vi "1.2odb.vi"() -> ()   [LabVIEW 2020]
panel:
  out "Waveform Chart":i32(graph)
  out "Numeric":i32
  in  "stop":bool
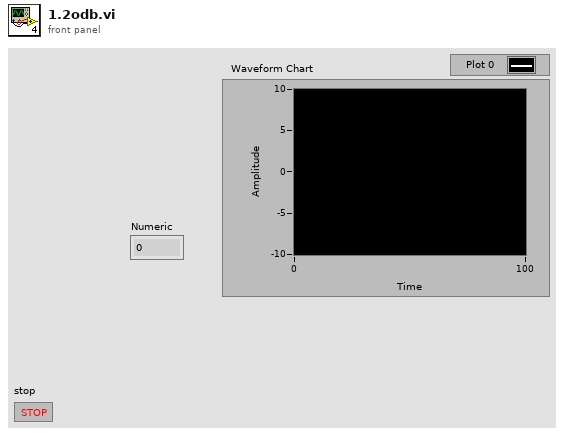
[diagram p1: front panel]
types:
  T1 = enum16{"Read", "Write", "ReadWrite", "BufferedRead", "BufferedReadWrite"}
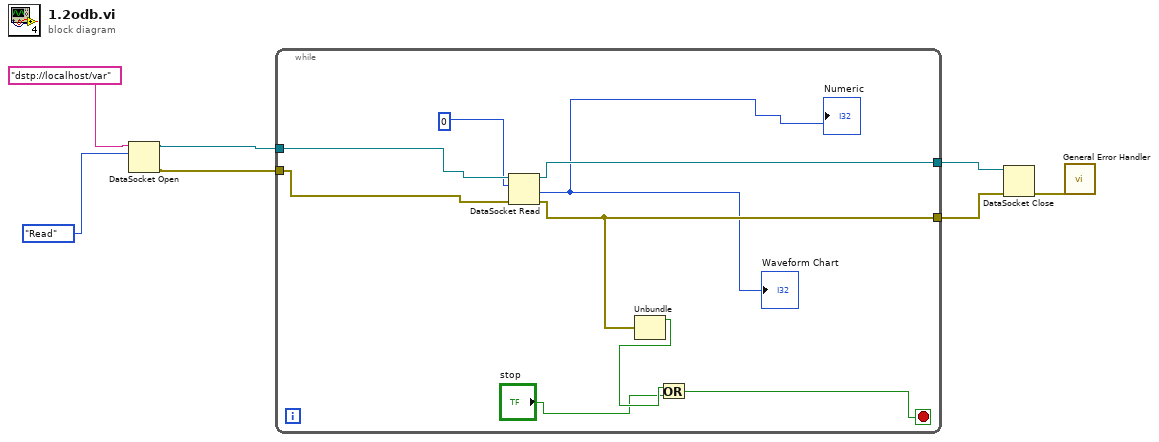
[diagram p0: block diagram]
diagram:
  n1 = DataSocket Open(10:T1."Read" ("mode"), 11:"dstp://localhost/var") -> (0:w5:errorcluster, 3:w6:refnum<k13>)  [unwired: 2 in]
  n2 = while {
    tunnel: w6 -> [w13]
    tunnel: w5 -> [w12]
    tunnel: [w10] -> w4
    tunnel: [w9] -> w3
    stop <- w14 stop-if-true
    n3 = DataSocket Read(8:w12, 10:0, 11:w13) -> (0:w9:errorcluster, 2:→"Numeric" →"Waveform Chart":i32, 3:w10:refnum<k13>)  [unwired: 2 in, 4 out]
    n4 = Unbundle(w9) -> ("status"=w16:bool)  [unwired: 2 out]
    n5 = Or(x=w16, y="stop") -> (x .or. y?=w14:bool)
  }
  n6 = DataSocket Close(8:w3, 11:w4) -> (0:w2:errorcluster)  [unwired: 1 in, 1 out]
  n7 = call <vilib>:"General Error Handler.vi"("error in (no error)"=w2) -> ()  [unwired: 10 in, 5 out]
